vi "DB Import Action - Create Chans.vi"(8 "error in (no error)":errorcluster, 10 "selected path":path, 11 "Node Ptr":u64) -> (0 "error out":errorcluster, 2 "selected path out":path caption="selected path", 3 "Node Ptr dup":u64)   [LabVIEW 2017, in "Ballard 1553 System Explorer.lvlib"]
uses:
  Ballard 1553 System Explorer.lvlib
  <vilib>/NI Veristand/Custom Device API/Set Item Property (Boolean).vi
  Create Sysdef Tree from DB Channel Clusters_RTs.vi
  Create Sysdef Tree from DB Channel Clusters_BC.vi
  <vilib>/NI Veristand/Custom Device API/NI VeriStand - Add Custom Device Section.vi
  Shared/Controls and Global/Global.vi
  <vilib>/NI VeriStand/Custom Device API/Custom Device API.lvlib
  Shared/Ballard 1553 Shared.lvlib
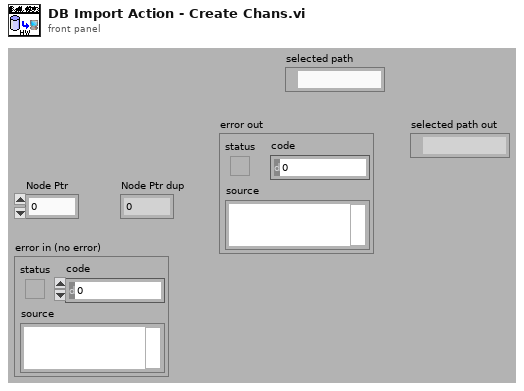
[diagram p1: front panel]
types:
  T1 = typedef "Ballard 1553 System Explorer.lvlib/Ballard_Channel.ctl" = cluster{"hardwareChannel":i32, "name":string, "BC":T2, "RTs":T10[], "ID":i32, "amplitudePercent":dbl}
  T2 = typedef "Ballard 1553 System Explorer.lvlib/Ballard_BC.ctl" = cluster{"ID":i32, "name":string, "messageBuffers":cluster{"ID":i32, "name":string, "messageData":u16[]}[], "messages":T3[], "minorFrames":T7[], "majorFrames":T8[], "acyclicFrames":T9[]}
  T3 = typedef "Ballard 1553 System Explorer.lvlib/Ballard_message.ctl" = cluster{"ID":i32, "name":string, "messageBufferIDRef":i32, "messageType":T4, "CWD1":T5, "CWD2":T6}
  T4 = typedef "Ballard 1553 System Explorer.lvlib/Ballard_messageType.ctl" = enum16{"BC to RT", "RT to BC", "RT to RT", "MC (Rx)", "MC (Tx)"}
  T5 = typedef "Ballard 1553 System Explorer.lvlib/Ballard_CWD1.ctl" = cluster{"TA (RT)":i8, "SA":i8, "Mode Code":i8, "Words Count":i8}
  T6 = typedef "Ballard 1553 System Explorer.lvlib/Ballard_CWD2.ctl" = cluster{"TA (RT)":i8, "SA":i8, "Words (WC)":i8}
  T7 = typedef "Ballard 1553 System Explorer.lvlib/Ballard_minorFrame.ctl" = cluster{"ID":i32, "name":string, "frameTime":i32, "messageIDRefs":i32[]}
  T8 = typedef "Ballard 1553 System Explorer.lvlib/Ballard_majorFrame.ctl" = cluster{"ID":i32, "name":string, "loopCount":i32, "minorFrameIDRef":i32[]}
  T9 = typedef "Ballard 1553 System Explorer.lvlib/Ballard_acyclicFrame.ctl" = cluster{"ID":i32, "name":string, "messageIDRefs":i32[]}
  T10 = typedef "Ballard 1553 System Explorer.lvlib/Ballard_RT.ctl" = cluster{"ID":i32, "name":string, "rtAddress":i8, "responseTime":i32, "messageBuffers":cluster{"ID":i32, "name":string, "messageData":u16[]}[], "subAddresses":T11[], "rtMode":T13, "initialSwd":u16}
  T11 = typedef "Ballard 1553 System Explorer.lvlib/Ballard_RT subAddress.ctl" = cluster{"ID":i32, "name":string, "messageBufferIDRef":i32, "subAddress":i8, "direction":T12}
  T12 = typedef "Ballard 1553 System Explorer.lvlib/Ballard_RT direction.ctl" = enum16{"Tx", "Rx"}
  T13 = typedef "Ballard 1553 System Explorer.lvlib/Ballard_RT rtMode.ctl" = enum16{"Simulate", "Monitor", "Disable"}
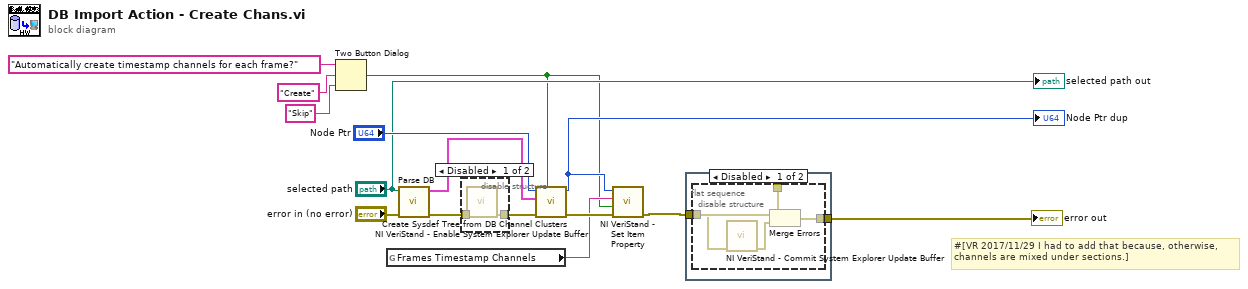
[diagram p0: block diagram]
diagram:
  # "#[VR 2017/11/29 I had to add that because, otherwise,\nchannels are mixed under sections.]"
  n1 = Two Button Dialog(message="Automatically create timestamp channels for each frame?", 1:"Skip" ("F button name (\"Cancel\")"), 2:"Create" ("T button name (\"OK\")")) -> (T button?=w2:bool)
  n2 = global read "Global.vi" "Frames Timestamp Channels"() -> (w3:string)
  n3 = call "Parse DB.vi"("error in (no error)"="error in (no error)", "Path in"="selected path") -> ("error out"=w7:errorcluster, "channels"=w14:T1[])  [unwired: 8 in]
  n4 = disable-structure shown="Disabled" {
    disable-tunnel: [w17 w18] -> w13
    disable-tunnel: w7 -> [w16 w18]
    frame Disabled {
      n5 = call <vilib>:"NI VeriStand - Enable System Explorer Update Buffer.vi"("error in (no error)"=w16) -> ("error out"=w17:errorcluster)  [unwired: 10 in]
    }
    frame Enabled {
    }
  }
  n6 = call "Create Sysdef Tree from DB Channel Clusters.vi"("Autocreate Rx timestamp chans?"=w2, "error in"=w13, "channels"=w14, "Device Ptr"="Node Ptr") -> ("error out"=w5:errorcluster, "Device Ptr dup"=w6:u64)  [unwired: 6 in]
  "Node Ptr dup" <- w6
  n7 = call-poly <vilib>:"NI VeriStand - Set Item Property.vi"("error in (no error)"=w5, "Value"=w2, "Property Name"=w3, "Item Ref in"=w6) -> ("error out"=w4:errorcluster)  [unwired: 5 in, 2 out]
  n8 = flat-sequence {
    tunnel: w4 -> [w19]
    tunnel: [w20] -> w1
    frame #0 {
      n9 = disable-structure shown="Disabled" {
        disable-tunnel: w19 -> [w24 _]
        disable-tunnel: [w22 w25] -> w20
        disable-tunnel: w19 -> [w21 w25]
        frame Disabled {
          n10 = call <vilib>:"NI VeriStand - Commit System Explorer Update Buffer.vi"("error in (no error)"=w21) -> ("error out"=w23:errorcluster)  [unwired: 10 in]
          n11 = Merge Errors(w24, w23) -> (w22:errorcluster)
        }
        frame Enabled {
        }
      }
    }
  }
  "error out" <- w1
  "selected path out" <- "selected path"
